vi "Reset.vi"(0 "VISA resource name":refnum<visa-resource-name>, 1 "Error Queue Option":enum16{"Clear Error Queue", "Error Query"}(ring), 11 "error in (no error)":errorcluster) -> (4 "VISA resource name out":refnum<visa-resource-name>, 15 "error out":errorcluster)   [LabVIEW 2014, in "KE6514Driver.lvlib"]
doc: "Resets the 622x and optionally clears the error queue."
uses:
  KE6514Driver.lvlib
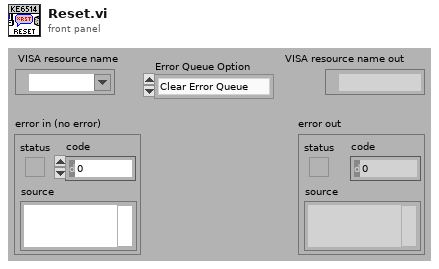
[diagram p1: front panel]
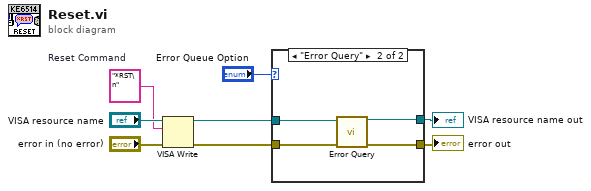
[diagram p0: block diagram]
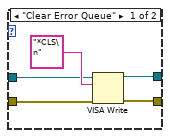
[diagram p2: hidden frame]
diagram:
  w6 = "*RST\n"  # Reset Command
  n1 = VISA Write(VISA resource name="VISA resource name", write buffer=w6, error in (no error)="error in (no error)") -> (VISA resource name out=w1:refnum<visa-resource-name>, error out=w2:errorcluster)  [unwired: 1 out]
  n2 = case shown="\"Error Query\"" "Error Queue Option" {
    tunnel: [w9 w17] -> w5
    tunnel: [w12 w16] -> w4
    tunnel: w2 -> [w13 w14]
    tunnel: w1 -> [w10 w15]
    frame "Clear Error Queue" {
      n3 = VISA Write(VISA resource name=w10, write buffer="*CLS\n", error in (no error)=w13) -> (VISA resource name out=w9:refnum<visa-resource-name>, error out=w12:errorcluster)  [unwired: 1 out]
    }
    frame "Error Query" {
      n4 = call "Error Query.vi"("VISA Resource In"=w15, "error in (no error)"=w14) -> ("VISA Resource Out (dupl)"=w17:refnum<visa-resource-name>, "error out"=w16:errorcluster)  [unwired: 10 in, 2 out]
    }
  }
  "error out" <- w4
  "VISA resource name out" <- w5
